vi "Forward.vi"(10 "Msg Attributes in":refnum<data-value>) -> (0 "Error out":errorcluster, 2 "Msg Attributes out":refnum<data-value>)   [LabVIEW 2020, in "_Template.lvlib" / "Templates.lvlib" / "TEMPLATE jettl Msg.lvlib"]
uses:
  TEMPLATE jettl Msg.lvlib
  jettl/jettl/Relation.ctl
  jettl/jettl/jettl.lvlib
  jettl/jettl/Teller.ctl
  jettl/jettl/Msg Input/Msg Input.lvclass
  jettl/jettl/Msg Output/Msg Output.lvclass
  jettl/jettl/Msg/Msg.lvclass
  jettl/jettl/Msg Attributes.ctl
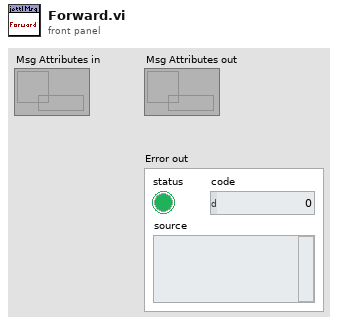
[diagram p1: front panel]
types:
  T1 = typedef "jettl.lvlib/Msg Attributes.ctl" = cluster{"Msg":refnum<class "Msg.lvclass">, "Msg Input":refnum<class "Msg Input.lvclass">, "Msg Output":refnum<class "Msg Output.lvclass">, "Teller":T2}
  T2 = typedef "jettl.lvlib/Teller.ctl" = cluster{"Absolute Time":timestamp, "Relative Time":dbl, "Alias":string, "Relation":T3}
  T3 = typedef "jettl.lvlib/Relation.ctl" = enum16{"Self", "Parent", "Child"}
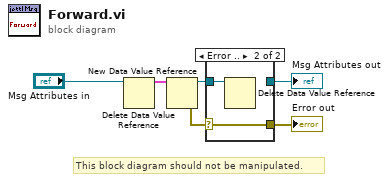
[diagram p0: block diagram]
diagram:
  # "This block diagram should not be manipulated."
  n1 = Delete Data Value Reference(data value reference="Msg Attributes in") -> (data value=w3:T1)  [unwired: 1 in, 1 out]
  n2 = New Data Value Reference(data value=w3) -> (data value reference=w5:refnum<data-value>, error out=w4:errorcluster)  [unwired: 1 in]
  n3 = case shown="Error .." w4 {
    selector: w4 -> [_ w8]
    tunnel: w5 -> [w7 w9]
    tunnel: [w7 _] -> w1
    tunnel: [_ w8] -> w2
    frame No Error {
    }
    frame Error {
      n4 = Delete Data Value Reference(data value reference=w9) -> ()  [unwired: 1 in, 2 out]
    }
  }
  "Error out" <- w2
  "Msg Attributes out" <- w1
